vi "Parse JSON String (LV).vi"(7 "Default Value":variant, 8 "error in (no error)":errorcluster, 11 "String":string) -> (0 "error out":errorcluster, 3 "Value":variant)   [LabVIEW 2015, in "JSON.lvlib"]
uses:
  JSON.lvlib
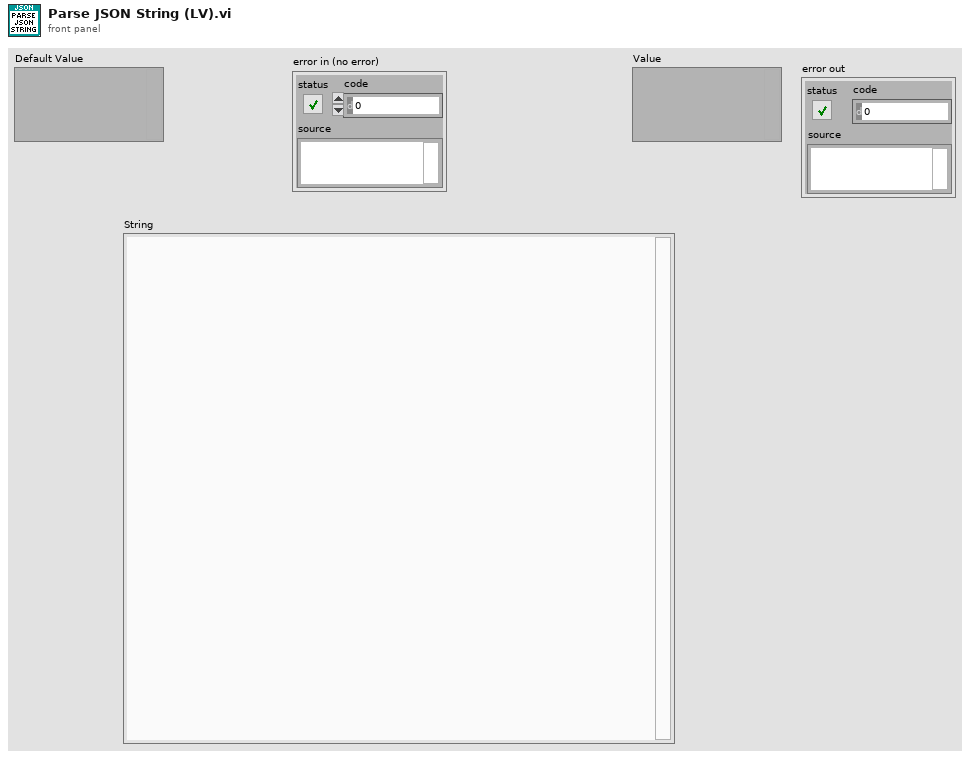
[diagram p1: front panel]
types:
  T1 = typedef "JSON.lvlib/JSON Value.ctl" = cluster{"\\type":enum16{"Object", "Array", "String", "Number", "Boolean", "Null"}, "ÿýÿýÿýÿýÿýÿþÿýÿýÿý#JSON.lvlib:JSON Name-Value Pair.ctlÿýÿýÿýÿýÿýÿþÿýÿýÿýJSON.lvlib:JSON Value.ctl":variant}
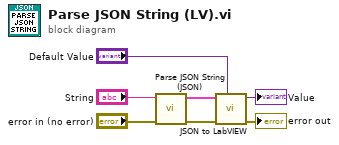
[diagram p0: block diagram]
diagram:
  n1 = call "Parse JSON String (JSON).vi"("error in (no error)"="error in (no error)", "String"="String") -> ("error out"=w3:errorcluster, "Value"=w7:T1)  [unwired: 8 in]
  n2 = call "JSON to LabVIEW.vi"("Default Value"="Default Value", "error in (no error)"=w3, "JSON Value"=w7) -> ("error out"=→"error out":errorcluster, "LV Value"=→"Value":variant)  [unwired: 7 in]
